vi "Main.vi"() -> ()   [LabVIEW 2024]
uses:
  Controls/Mode Enums/Bipolar Enum.ctl
  Controls/Activate Bools/Bipolar Activate Bool.ctl
  Controls/Plus-Minus Bools/Bipolar plus Bool.ctl
  Controls/Plus-Minus Bools/Bipolar minus Bool.ctl
  Controls/Activate Bools/Ligasure Activate Bool.ctl
  Controls/Mode Enums/Mono2 Coag Enum.ctl
  Controls/Activate Bools/Mono2 Coag Activate Bool.ctl
  Controls/Plus-Minus Bools/Mono2 Coag plus Bool.ctl
  Controls/Plus-Minus Bools/Mono2 Coag minus Bool.ctl
  Controls/Mode Enums/Mono2 Cut Enum.ctl
  Controls/Activate Bools/Mono2 Cut Activate Bool.ctl
  Controls/Plus-Minus Bools/Mono2 Cut plus Bool.ctl
  Controls/Plus-Minus Bools/Mono2 Cut minus Bool.ctl
  Controls/Mode Enums/Mono1 Coag Enum.ctl
  Controls/Activate Bools/Mono1 Coag Activate Bool.ctl
  Controls/Plus-Minus Bools/Mono1 Coag minus Bool.ctl
  Controls/Plus-Minus Bools/Mono1 Coag plus Bool.ctl
  Controls/Activate Bools/Mono1 Cut Activate Bool.ctl
  Controls/Mode Enums/Mono1 Cut Enum.ctl
  Controls/Plus-Minus Bools/Mono1 Cut plus Bool.ctl
  Controls/Plus-Minus Bools/Mono1 Cut minus Bool.ctl
  Controls/Tab Enums/Mono1 - Tab.ctl
  Controls/Tab Enums/Mono2 - Tab.ctl
  Controls/Activate Bools/Mono2 Triverse Activate Bool.ctl
  Controls/Tab Enums/Ligasure - Tab.ctl
  Controls/Tab Enums/Bipolar - Tab.ctl
  Controls/Cntrl - Power Bool.ctl
  Controls/QMH Fundamentals - Message Cluster.ctl
  Controls/Clusters/Message Handling Cluster.ctl
  Controls/Clusters/Control Handling Cluster.ctl
  Controls/Tab Enums/Activation Type Enum.ctl
  Controls/Clusters/Change Power Level Cluster.ctl
  Controls/Clusters/Activate Port Cluster.ctl
  Controls/Clusters/Change Mode Cluster.ctl
panel:
  in  "Show Graph":bool
  out "Display Message":string
  in  "Logging":bool
  in  "Power":T1
  in  "Main Tab":T2(tab)
  in  "CSV Test Path":path
  in  "Test Tab":enum32{"Run Test", "Edit Test"}(tab)
  in  "Abort Test":bool
  in  "Run Test":bool
  in  "Save CSV":bool
  in  "BldScript":i32[](listbox)
  in  "Load CSV":bool
  in  "Bipolar Enum":T3
  in  "Bipolar Activate":T4
  in  "Bipolar plus":T5
  in  "Bipolar minus":T6
  out "Bipolar Power":string
  in  "Ligasure Activate":T7
  in  "Mono2 Coag Enum":T8
  in  "Mono2 Coag Activate":T9
  in  "Mono2 Coag minus":T10
  in  "Mono2 Cut Enum":T11
  in  "Mono2 Cut Activate":T12
  in  "Mono2 Cut plus":T13
  in  "Mono2 Cut minus":T14
  out "Mono2 - Coag Power":string
  out "Mono2 - Cut Power":string
  in  "Mono2 Coag plus":T15
  in  "Mono1 Coag Enum":T16
  in  "Mono1 Coag Activate":T17
  in  "Mono1 Coag minus":T18
  in  "Mono1 Coag plus":T19
  out "Mono1 - Coag Power":string
  in  "Mono1 Cut Activate":T20
  out "Mono1 - Cut Power":string
  in  "Mono1 Cut Enum":T21
  in  "Mono1 Cut plus":T22
  in  "Mono1 Cut minus":T23
  in  "Mono1 - Tab":T24
  in  "Mono2 - Tab":T25
  in  "Mono2 Triverse Slide":i8(slide)=1 scale=1.0..5.0
  in  "Mono2 Triverse Activate":T26
  in  "Ligasure - Tab":T27
  in  "Bipolar - Tab":T28=enum."Auto Bipolar"
  in  "Connections Tab":T29(tab)
  in  "S2C Tab":enum32{"Build Script", "Execute Script"}(tab)
  in  "BldScript 2":i32[](listbox)
  in  "SubScript":string caption="SubScript Filename"
  in  "BldScriptFile":path caption="Test Script File"
  in  "BldBack":bool
  in  "BldLoadScript":bool
  in  "BldSaveScript":bool
  in  "BldSaveScriptAs":bool
  in  "BldClear":bool
  in  "ExeLoadScript":bool
  in  "ExeScriptFile":path caption="Script File"
  in  "ExeScript":i32[](listbox)
  in  "ExeExecute":bool
  in  "ExePause":bool
  in  "ExeNext":bool
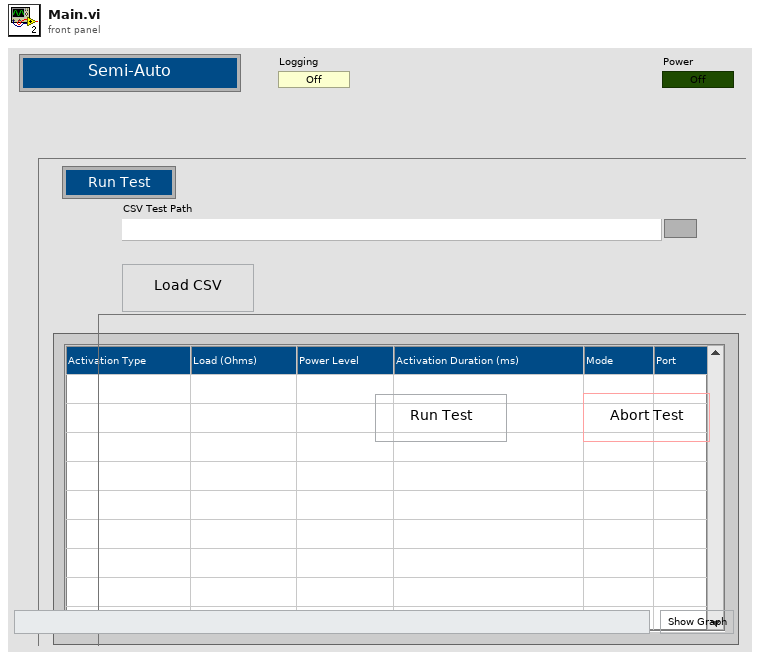
[diagram p1: front panel]
types:
  T1 = typedef "Cntrl - Power Bool.ctl" = bool
  T2 = enum32{"Semi-Auto", "Manual", "Connections", "Script 2 Code"}
  T3 = typedef "Bipolar Enum.ctl" = enum16{"Standard", "Macro", "Precision"}
  T4 = typedef "Bipolar Activate Bool.ctl" = bool
  T5 = typedef "Bipolar plus Bool.ctl" = bool
  T6 = typedef "Bipolar minus Bool.ctl" = bool
  T7 = typedef "Ligasure Activate Bool.ctl" = bool
  T8 = typedef "Mono2 Coag Enum.ctl" = enum16{"Spray", "Fulgerate"}
  T9 = typedef "Mono2 Coag Activate Bool.ctl" = bool
  T10 = typedef "Mono2 Coag minus Bool.ctl" = bool
  T11 = typedef "Mono2 Cut Enum.ctl" = enum16{"Pure", "Blend"}
  T12 = typedef "Mono2 Cut Activate Bool.ctl" = bool
  T13 = typedef "Mono2 Cut plus Bool.ctl" = bool
  T14 = typedef "Mono2 Cut minus Bool.ctl" = bool
  T15 = typedef "Mono2 Coag plus Bool.ctl" = bool
  T16 = typedef "Mono1 Coag Enum.ctl" = enum16{"Spray", "Fulgerate"}
  T17 = typedef "Mono1 Coag Activate Bool.ctl" = bool
  T18 = typedef "Mono1 Coag minus Bool.ctl" = bool
  T19 = typedef "Mono1 Coag plus Bool.ctl" = bool
  T20 = typedef "Mono1 Cut Activate Bool.ctl" = bool
  T21 = typedef "Mono1 Cut Enum.ctl" = enum16{"Pure", "Blend"}
  T22 = typedef "Mono1 Cut plus Bool.ctl" = bool
  T23 = typedef "Mono1 Cut minus Bool.ctl" = bool
  T24 = typedef "Mono1 - Tab.ctl" = enum32{"Mono1 - Fornax", "Mono1 - Handswitch", "Mono1 - Footswitch"}
  T25 = typedef "Mono2 - Tab.ctl" = enum32{"Mono2 - Fornax", "Mono2 - Handswitch", "Mono2 - Footswitch", "Mono2 - Triverse"}
  T26 = typedef "Mono2 Triverse Activate Bool.ctl" = bool
  T27 = typedef "Ligasure - Tab.ctl" = enum32{"Ligasure - Fornax", "Ligasure - Handswitch", "Ligasure - Footswitch"}
  T28 = typedef "Bipolar - Tab.ctl" = enum32{"Bipolar - Fornax", "Bipolar - Handswitch", "Bipolar - Footswitch", "Auto Bipolar"}
  T29 = enum32{"Digitizer Tab", "Fornax Tab", "FPGA Tab", "Nike Tab", "Relay Tab", "Rigel Tab"}
  T30 = typedef "Control Handling Cluster.ctl" = cluster{"Mono1 - Tab Enum":T31, "Mono2 - Tab Enum":T31, "Bipolar - Tab Enum":T31, "Ligasure - Tab Enum":T31}
  T31 = typedef "Activation Type Enum.ctl" = enum16{"Fornax", "Handswitch", "Footswitch", "Triverse", "Auto Bipolar"}
  T32 = typedef "Message Handling Cluster.ctl" = cluster{"Boolean":bool}
  T33 = typedef "QMH Fundamentals - Message Cluster.ctl" = cluster{"Message":string, "Message Data":variant}
  T34 = enum16{"Mono1 Cut", "Mono1 Coag", "Mono2 Cut", "Mono2 Coag", "Bipolar"}
  T35 = typedef "Change Power Level Cluster.ctl" = cluster{"Activation Type":enum16{"Mono1 Cut", "Mono1 Coag", "Mono2 Cut", "Mono2 Coag", "Bipolar"}, "Plus-Minus":enum16{"Plus", "Minus"}, "Plus-Minus":bool}
  T36 = enum16{"Mono1 Cut", "Mono1 Coag", "Mono2 Cut", "Mono2 Coag", "Mono2 Triverse", "Bipolar", "Ligasure"}
  T37 = typedef "Activate Port Cluster.ctl" = cluster{"Port":enum16{"Mono1 Cut", "Mono1 Coag", "Mono2 Cut", "Mono2 Coag", "Mono2 Triverse", "Bipolar", "Ligasure"}, "Activation Type Enum":T31, "Activate/Deactivate":bool}
  T38 = enum16{"Mono1 - Tab", "Mono2 - Tab", "Bipolar - Tab", "Ligasure - Tab"}
  T39 = enum32{"Invalid", "Standard", "Closed", "Hidden", "Minimized", "Maximized"}
  T40 = typedef "Change Mode Cluster.ctl" = cluster{"Port":enum16{"Mono1", "Mono2", "Bipolar", "Ligasure"}, "Mode":enum16{"Mono Pure", "Mono Blend", "Mono Fulgerate", "Mono Spray", "Bi Precision", "Bi Macro", "Bi Standard"}}
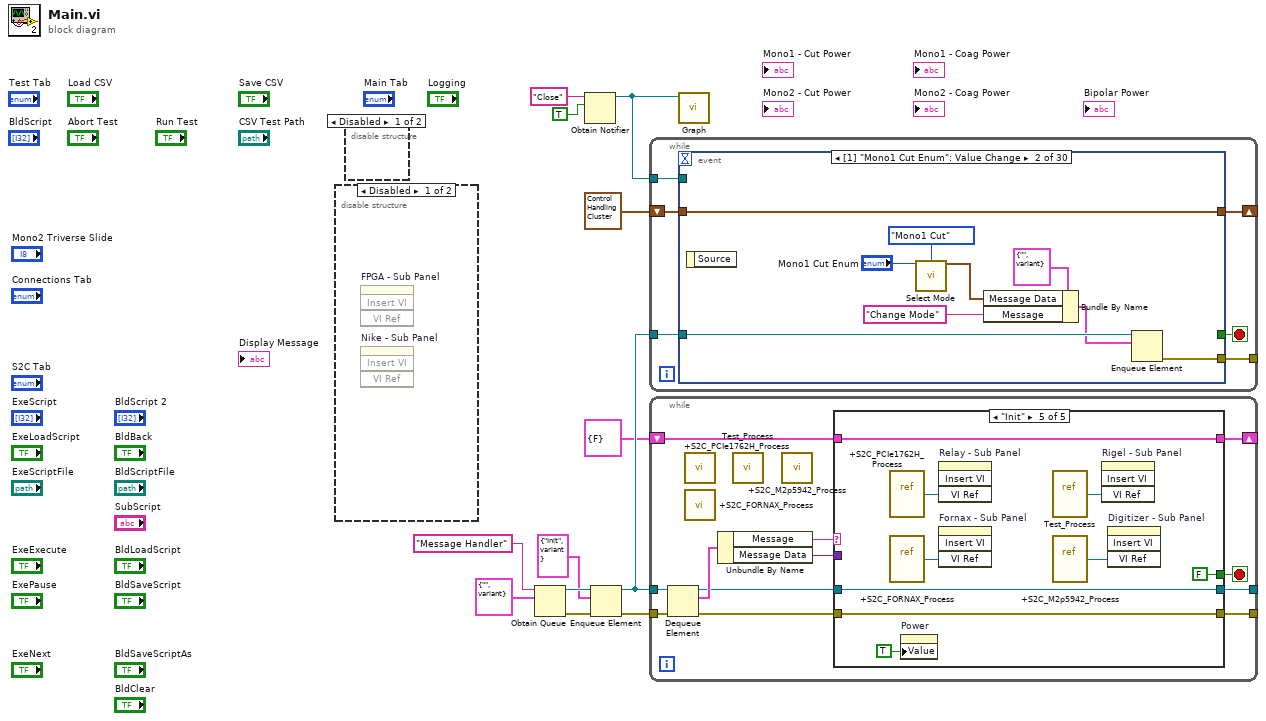
[diagram p0: block diagram]
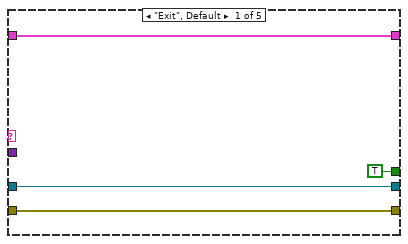
[diagram p4: hidden frame]
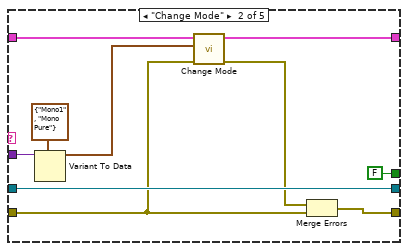
[diagram p5: hidden frame]
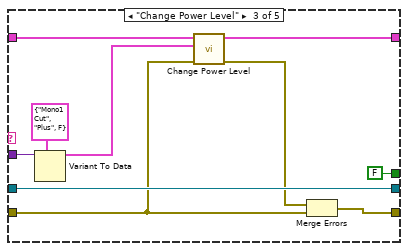
[diagram p6: hidden frame]
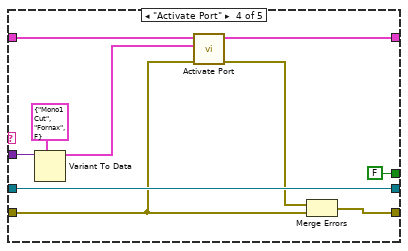
[diagram p7: hidden frame]
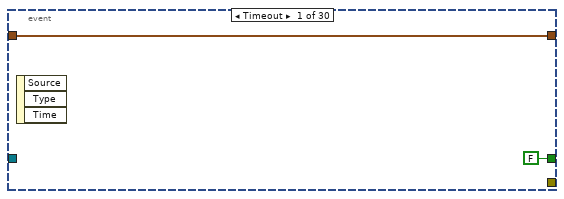
[diagram p8: hidden frame]
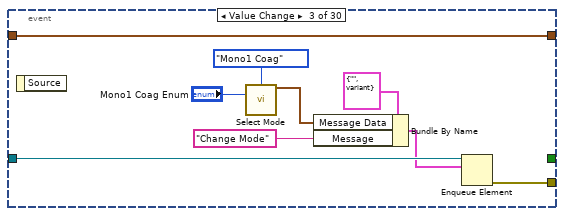
[diagram p9: hidden frame]
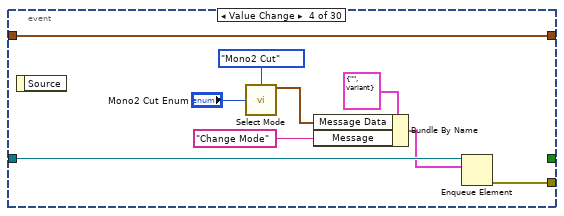
[diagram p10: hidden frame]
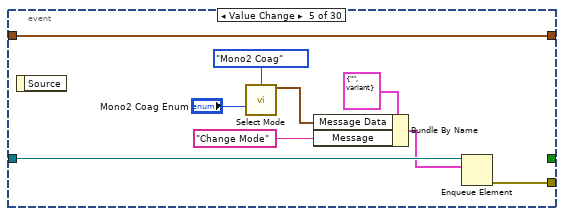
[diagram p11: hidden frame]
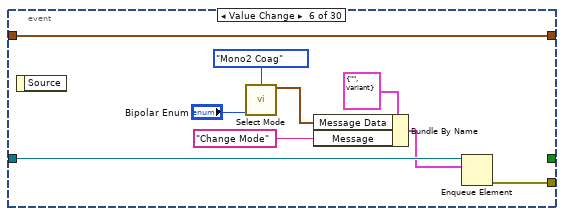
[diagram p12: hidden frame]
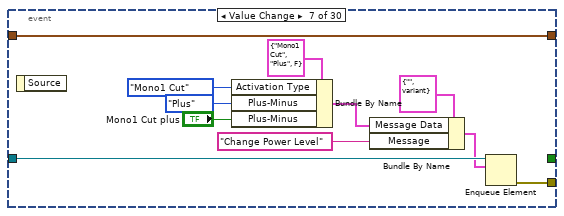
[diagram p13: hidden frame]
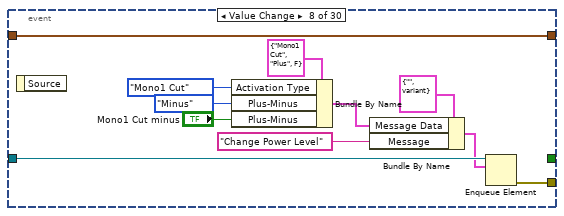
[diagram p14: hidden frame]
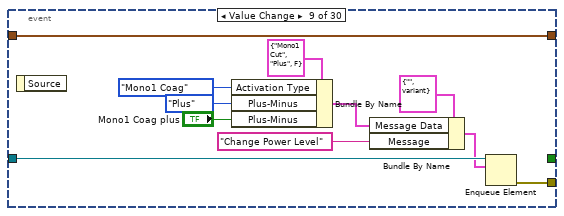
[diagram p15: hidden frame]
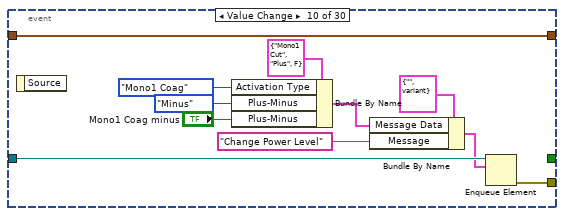
[diagram p16: hidden frame]
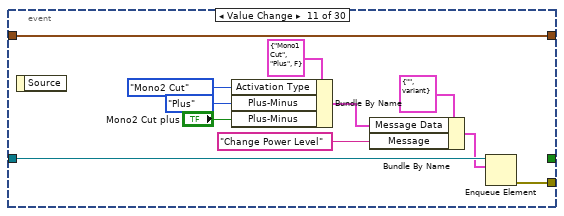
[diagram p17: hidden frame]
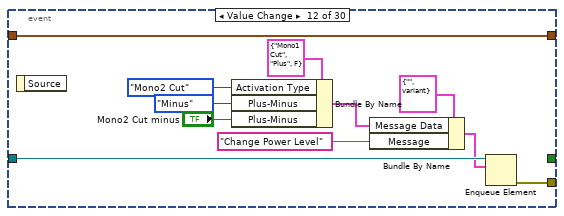
[diagram p18: hidden frame]
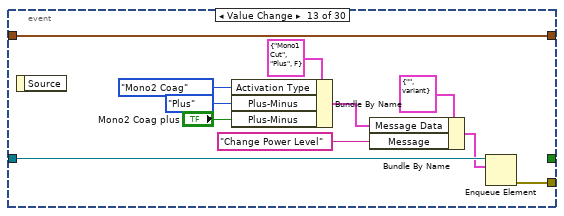
[diagram p19: hidden frame]
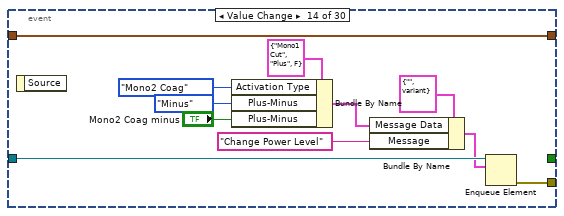
[diagram p20: hidden frame]
diagram:
  n1 = disable-structure shown="Disabled" {
    frame Disabled {
      n2 = invoke on="FPGA - Sub Panel" class="SubPnl" method="Insert VI"() -> ()  [unwired: 4 in, 4 out]
      n3 = invoke on="Nike - Sub Panel" class="SubPnl" method="Insert VI"() -> ()  [unwired: 4 in, 4 out]
    }
    frame Enabled {
    }
  }
  n4 = disable-structure shown="Disabled" {
    frame Disabled {
    }
    frame Enabled {
    }
  }
  n5 = Obtain Queue(name (unnamed)="Message Handler", element data type=T33 {"Message"="", "Message Data"=variant} ("Message Cluster")) -> (queue out=w11:refnum<queue>, error out=w12:errorcluster)  [unwired: 3 in, 1 out]
  n6 = Obtain Notifier(name (unnamed)="Close", notification data type=TRUE) -> (notifier out=w1:refnum<notifier>)  [unwired: 2 in, 2 out]
  n7 = Enqueue Element(queue=w11, element=T33 {"Message"="Init", "Message Data"=variant} ("Message Cluster"), error in (no error)=w12) -> (queue out=w6:refnum<queue>, error out=w9:errorcluster)  [unwired: 1 in, 1 out]
  n8 = while {
    tunnel: w6 -> [w17]
    tunnel: [w16] -> _
    shift-right: [w15] -> _
    shift-left: T30 {"Mono1 - Tab Enum"=enum."Fornax", "Mono2 - Tab Enum"=enum."Fornax", "Bipolar - Tab Enum"=enum."Fornax", "Ligasure - Tab Enum"=enum."Fornax"} ("Control Handling Cluster") -> [w14]
    tunnel: w1 -> [w13]
    stop <- w18 stop-if-true
    n9 = event shown="[1] \"Mono1 Cut Enum\": Value Change" {
      selector: _ -> [_ _ _ _ _ _ _ _ _ _ _ _ _ _ _ _ _ _ _ _ _ _ _ _ _ _ _ _ _ _]
      dyn-events: _ -> [_ _ _ _ _ _ _ _ _ _ _ _ _ _ _ _ _ _ _ _ _ _ _ _ _ _ _ _ _ _]
      timeout: _ -> [_ _ _ _ _ _ _ _ _ _ _ _ _ _ _ _ _ _ _ _ _ _ _ _ _ _ _ _ _ _]
      tunnel: [FALSE _ _ _ _ _ _ _ _ _ _ _ _ _ _ _ _ _ _ _ _ _ _ _ _ _ _ _ TRUE w286] -> w18
      tunnel: w17 -> [_ w29 w38 w47 w56 w65 w76 w87 w98 w109 w120 w131 w142 w153 w164 w175 w178 w190 w201 w212 w223 w234 w245 _ _ _ _ _ w285 w292]
      tunnel: [_ w26 w35 w44 w53 w62 w73 w84 w95 w106 w117 w128 w139 w150 w161 w172 w176 w188 w199 w210 w221 w232 w243 _ _ _ _ _ w283 w290] -> w16
      tunnel: [w19 w21 w30 w39 w48 w57 w71 w82 w93 w104 w115 w126 w137 w148 w159 w170 w185 w196 w207 w218 w229 w240 w251 w254 w260 w265 w270 w273 w281 w289] -> w15
      tunnel: w14 -> [w19 w21 w30 w39 w48 w57 w71 w82 w93 w104 w115 w126 w137 w148 w159 w170 w185 w196 w207 w218 w229 w240 w251 w257 w262 w267 w272 w273 w281 w289]
      tunnel: w13 -> [_ _ _ _ _ _ _ _ _ _ _ _ _ _ _ _ _ _ _ _ _ _ _ _ _ _ _ _ w279 w287]
      event Timeout {
        n10 = event-data() -> ()  [unwired: 1 in, 3 out]
      }
      event Value Change {
        n11 = event-data() -> ()  [unwired: 1 in, 1 out]
        n12 = call "Select Mode.vi"("Mono1 Cut Enum"="Mono1 Cut Enum", "Activation Type"=T34."Mono1 Cut") -> ("Change Mode Cluster"=w24:T40)  [unwired: 13 in]
        n13 = Bundle By Name(cluster=T33 {"Message"="", "Message Data"=variant} ("Message Cluster"), "Message Data"=w24, "Message"="Change Mode") -> (w27:T33)
        n14 = Enqueue Element(queue=w29, element=w27) -> (error out=w26:errorcluster)  [unwired: 2 in, 2 out]
      }
      event Value Change {
        n15 = event-data() -> ()  [unwired: 1 in, 1 out]
        n16 = call "Select Mode.vi"("Activation Type"=T34."Mono1 Coag", "Mono1 Coag Enum"="Mono1 Coag Enum") -> ("Change Mode Cluster"=w33:T40)  [unwired: 13 in]
        n17 = Bundle By Name(cluster=T33 {"Message"="", "Message Data"=variant} ("Message Cluster"), "Message Data"=w33, "Message"="Change Mode") -> (w36:T33)
        n18 = Enqueue Element(queue=w38, element=w36) -> (error out=w35:errorcluster)  [unwired: 2 in, 2 out]
      }
      event Value Change {
        n19 = event-data() -> ()  [unwired: 1 in, 1 out]
        n20 = call "Select Mode.vi"("Activation Type"=T34."Mono2 Cut", "Mono2 Cut Enum"="Mono2 Cut Enum") -> ("Change Mode Cluster"=w42:T40)  [unwired: 13 in]
        n21 = Bundle By Name(cluster=T33 {"Message"="", "Message Data"=variant} ("Message Cluster"), "Message Data"=w42, "Message"="Change Mode") -> (w45:T33)
        n22 = Enqueue Element(queue=w47, element=w45) -> (error out=w44:errorcluster)  [unwired: 2 in, 2 out]
      }
      event Value Change {
        n23 = event-data() -> ()  [unwired: 1 in, 1 out]
        n24 = call "Select Mode.vi"("Activation Type"=T34."Mono2 Coag", "Mono2 Coag Enum"="Mono2 Coag Enum") -> ("Change Mode Cluster"=w51:T40)  [unwired: 13 in]
        n25 = Bundle By Name(cluster=T33 {"Message"="", "Message Data"=variant} ("Message Cluster"), "Message Data"=w51, "Message"="Change Mode") -> (w54:T33)
        n26 = Enqueue Element(queue=w56, element=w54) -> (error out=w53:errorcluster)  [unwired: 2 in, 2 out]
      }
      event Value Change {
        n27 = event-data() -> ()  [unwired: 1 in, 1 out]
        n28 = call "Select Mode.vi"("Activation Type"=T34."Mono2 Coag", "Bipolar Enum"="Bipolar Enum") -> ("Change Mode Cluster"=w60:T40)  [unwired: 13 in]
        n29 = Bundle By Name(cluster=T33 {"Message"="", "Message Data"=variant} ("Message Cluster"), "Message Data"=w60, "Message"="Change Mode") -> (w63:T33)
        n30 = Enqueue Element(queue=w65, element=w63) -> (error out=w62:errorcluster)  [unwired: 2 in, 2 out]
      }
      event Value Change {
        n31 = event-data() -> ()  [unwired: 1 in, 1 out]
        n32 = Bundle By Name(cluster=T35 {"Activation Type"=enum."Mono1 Cut", "Plus-Minus"=enum."Plus", "Plus-Minus"=FALSE}, "Activation Type"=T34."Mono1 Cut", "Plus-Minus"=enum16{"Plus", "Minus"}."Plus", "Plus-Minus"="Mono1 Cut plus") -> (w67:T35)
        n33 = Bundle By Name(cluster=T33 {"Message"="", "Message Data"=variant} ("Message Cluster"), "Message Data"=w67, "Message"="Change Power Level") -> (w74:T33)
        n34 = Enqueue Element(queue=w76, element=w74) -> (error out=w73:errorcluster)  [unwired: 2 in, 2 out]
      }
      event Value Change {
        n35 = event-data() -> ()  [unwired: 1 in, 1 out]
        n36 = Bundle By Name(cluster=T35 {"Activation Type"=enum."Mono1 Cut", "Plus-Minus"=enum."Plus", "Plus-Minus"=FALSE}, "Activation Type"=T34."Mono1 Cut", "Plus-Minus"=enum16{"Plus", "Minus"}."Minus", "Plus-Minus"="Mono1 Cut minus") -> (w78:T35)
        n37 = Bundle By Name(cluster=T33 {"Message"="", "Message Data"=variant} ("Message Cluster"), "Message Data"=w78, "Message"="Change Power Level") -> (w85:T33)
        n38 = Enqueue Element(queue=w87, element=w85) -> (error out=w84:errorcluster)  [unwired: 2 in, 2 out]
      }
      event Value Change {
        n39 = event-data() -> ()  [unwired: 1 in, 1 out]
        n40 = Bundle By Name(cluster=T35 {"Activation Type"=enum."Mono1 Cut", "Plus-Minus"=enum."Plus", "Plus-Minus"=FALSE}, "Activation Type"=T34."Mono1 Coag", "Plus-Minus"=enum16{"Plus", "Minus"}."Plus", "Plus-Minus"="Mono1 Coag plus") -> (w89:T35)
        n41 = Bundle By Name(cluster=T33 {"Message"="", "Message Data"=variant} ("Message Cluster"), "Message Data"=w89, "Message"="Change Power Level") -> (w96:T33)
        n42 = Enqueue Element(queue=w98, element=w96) -> (error out=w95:errorcluster)  [unwired: 2 in, 2 out]
      }
      event Value Change {
        n43 = event-data() -> ()  [unwired: 1 in, 1 out]
        n44 = Bundle By Name(cluster=T35 {"Activation Type"=enum."Mono1 Cut", "Plus-Minus"=enum."Plus", "Plus-Minus"=FALSE}, "Activation Type"=T34."Mono1 Coag", "Plus-Minus"=enum16{"Plus", "Minus"}."Minus", "Plus-Minus"="Mono1 Coag minus") -> (w100:T35)
        n45 = Bundle By Name(cluster=T33 {"Message"="", "Message Data"=variant} ("Message Cluster"), "Message Data"=w100, "Message"="Change Power Level") -> (w107:T33)
        n46 = Enqueue Element(queue=w109, element=w107) -> (error out=w106:errorcluster)  [unwired: 2 in, 2 out]
      }
      event Value Change {
        n47 = event-data() -> ()  [unwired: 1 in, 1 out]
        n48 = Bundle By Name(cluster=T35 {"Activation Type"=enum."Mono1 Cut", "Plus-Minus"=enum."Plus", "Plus-Minus"=FALSE}, "Activation Type"=T34."Mono2 Cut", "Plus-Minus"=enum16{"Plus", "Minus"}."Plus", "Plus-Minus"="Mono2 Cut plus") -> (w111:T35)
        n49 = Bundle By Name(cluster=T33 {"Message"="", "Message Data"=variant} ("Message Cluster"), "Message Data"=w111, "Message"="Change Power Level") -> (w118:T33)
        n50 = Enqueue Element(queue=w120, element=w118) -> (error out=w117:errorcluster)  [unwired: 2 in, 2 out]
      }
      event Value Change {
        n51 = event-data() -> ()  [unwired: 1 in, 1 out]
        n52 = Bundle By Name(cluster=T35 {"Activation Type"=enum."Mono1 Cut", "Plus-Minus"=enum."Plus", "Plus-Minus"=FALSE}, "Activation Type"=T34."Mono2 Cut", "Plus-Minus"=enum16{"Plus", "Minus"}."Minus", "Plus-Minus"="Mono2 Cut minus") -> (w122:T35)
        n53 = Bundle By Name(cluster=T33 {"Message"="", "Message Data"=variant} ("Message Cluster"), "Message Data"=w122, "Message"="Change Power Level") -> (w129:T33)
        n54 = Enqueue Element(queue=w131, element=w129) -> (error out=w128:errorcluster)  [unwired: 2 in, 2 out]
      }
      event Value Change {
        n55 = event-data() -> ()  [unwired: 1 in, 1 out]
        n56 = Bundle By Name(cluster=T35 {"Activation Type"=enum."Mono1 Cut", "Plus-Minus"=enum."Plus", "Plus-Minus"=FALSE}, "Activation Type"=T34."Mono2 Coag", "Plus-Minus"=enum16{"Plus", "Minus"}."Plus", "Plus-Minus"="Mono2 Coag plus") -> (w133:T35)
        n57 = Bundle By Name(cluster=T33 {"Message"="", "Message Data"=variant} ("Message Cluster"), "Message Data"=w133, "Message"="Change Power Level") -> (w140:T33)
        n58 = Enqueue Element(queue=w142, element=w140) -> (error out=w139:errorcluster)  [unwired: 2 in, 2 out]
      }
      event Value Change {
        n59 = event-data() -> ()  [unwired: 1 in, 1 out]
        n60 = Bundle By Name(cluster=T35 {"Activation Type"=enum."Mono1 Cut", "Plus-Minus"=enum."Plus", "Plus-Minus"=FALSE}, "Activation Type"=T34."Mono2 Coag", "Plus-Minus"=enum16{"Plus", "Minus"}."Minus", "Plus-Minus"="Mono2 Coag minus") -> (w144:T35)
        n61 = Bundle By Name(cluster=T33 {"Message"="", "Message Data"=variant} ("Message Cluster"), "Message Data"=w144, "Message"="Change Power Level") -> (w151:T33)
        n62 = Enqueue Element(queue=w153, element=w151) -> (error out=w150:errorcluster)  [unwired: 2 in, 2 out]
      }
      event Value Change {
        n63 = event-data() -> ()  [unwired: 1 in, 1 out]
        n64 = Bundle By Name(cluster=T35 {"Activation Type"=enum."Mono1 Cut", "Plus-Minus"=enum."Plus", "Plus-Minus"=FALSE}, "Activation Type"=T34."Bipolar", "Plus-Minus"=enum16{"Plus", "Minus"}."Plus", "Plus-Minus"="Bipolar plus") -> (w155:T35)
        n65 = Bundle By Name(cluster=T33 {"Message"="", "Message Data"=variant} ("Message Cluster"), "Message Data"=w155, "Message"="Change Power Level") -> (w162:T33)
        n66 = Enqueue Element(queue=w164, element=w162) -> (error out=w161:errorcluster)  [unwired: 2 in, 2 out]
      }
      event Value Change {
        n67 = event-data() -> ()  [unwired: 1 in, 1 out]
        n68 = Bundle By Name(cluster=T35 {"Activation Type"=enum."Mono1 Cut", "Plus-Minus"=enum."Plus", "Plus-Minus"=FALSE}, "Activation Type"=T34."Bipolar", "Plus-Minus"=enum16{"Plus", "Minus"}."Minus", "Plus-Minus"="Bipolar minus") -> (w166:T35)
        n69 = Bundle By Name(cluster=T33 {"Message"="", "Message Data"=variant} ("Message Cluster"), "Message Data"=w166, "Message"="Change Power Level") -> (w173:T33)
        n70 = Enqueue Element(queue=w175, element=w173) -> (error out=w172:errorcluster)  [unwired: 2 in, 2 out]
      }
      event Value Change {
        n71 = event-data() -> ()  [unwired: 1 in, 1 out]
        n72 = Unbundle By Name(w185) -> ("Mono1 - Tab Enum"=w184:T31)
        n73 = Bundle By Name(cluster=T37 {"Port"=enum."Mono1 Cut", "Activation Type Enum"=enum."Fornax", "Activate/Deactivate"=FALSE}, "Activation Type Enum"=w184, "Port"=T36."Mono1 Cut", "Activate/Deactivate"="Mono1 Cut Activate") -> (w177:T37)
        n74 = Bundle By Name(cluster=T33 {"Message"="", "Message Data"=variant} ("Message Cluster"), "Message Data"=w177, "Message"="Activate Port") -> (w180:T33)
        n75 = Enqueue Element(queue=w178, element=w180) -> (error out=w176:errorcluster)  [unwired: 2 in, 2 out]
      }
      event Value Change {
        n76 = event-data() -> ()  [unwired: 1 in, 1 out]
        n77 = Unbundle By Name(w196) -> ("Mono1 - Tab Enum"=w195:T31)
        n78 = Bundle By Name(cluster=T37 {"Port"=enum."Mono1 Cut", "Activation Type Enum"=enum."Fornax", "Activate/Deactivate"=FALSE}, "Activation Type Enum"=w195, "Port"=T36."Mono1 Coag", "Activate/Deactivate"="Mono1 Coag Activate") -> (w189:T37)
        n79 = Bundle By Name(cluster=T33 {"Message"="", "Message Data"=variant} ("Message Cluster"), "Message Data"=w189, "Message"="Activate Port") -> (w192:T33)
        n80 = Enqueue Element(queue=w190, element=w192) -> (error out=w188:errorcluster)  [unwired: 2 in, 2 out]
      }
      event Value Change {
        n81 = event-data() -> ()  [unwired: 1 in, 1 out]
        n82 = Unbundle By Name(w207) -> ("Mono2 - Tab Enum"=w206:T31)
        n83 = Bundle By Name(cluster=T37 {"Port"=enum."Mono1 Cut", "Activation Type Enum"=enum."Fornax", "Activate/Deactivate"=FALSE}, "Activation Type Enum"=w206, "Port"=T36."Mono2 Cut", "Activate/Deactivate"="Mono2 Cut Activate") -> (w200:T37)
        n84 = Bundle By Name(cluster=T33 {"Message"="", "Message Data"=variant} ("Message Cluster"), "Message Data"=w200, "Message"="Activate Port") -> (w203:T33)
        n85 = Enqueue Element(queue=w201, element=w203) -> (error out=w199:errorcluster)  [unwired: 2 in, 2 out]
      }
      event Value Change {
        n86 = event-data() -> ()  [unwired: 1 in, 1 out]
        n87 = Unbundle By Name(w218) -> ("Mono2 - Tab Enum"=w217:T31)
        n88 = Bundle By Name(cluster=T37 {"Port"=enum."Mono1 Cut", "Activation Type Enum"=enum."Fornax", "Activate/Deactivate"=FALSE}, "Activation Type Enum"=w217, "Port"=T36."Mono2 Coag", "Activate/Deactivate"="Mono2 Coag Activate") -> (w211:T37)
        n89 = Bundle By Name(cluster=T33 {"Message"="", "Message Data"=variant} ("Message Cluster"), "Message Data"=w211, "Message"="Activate Port") -> (w214:T33)
        n90 = Enqueue Element(queue=w212, element=w214) -> (error out=w210:errorcluster)  [unwired: 2 in, 2 out]
      }
      event Value Change {
        n91 = event-data() -> ()  [unwired: 1 in, 1 out]
        n92 = Unbundle By Name(w229) -> ("Mono2 - Tab Enum"=w228:T31)
        n93 = Bundle By Name(cluster=T37 {"Port"=enum."Mono1 Cut", "Activation Type Enum"=enum."Fornax", "Activate/Deactivate"=FALSE}, "Activation Type Enum"=w228, "Port"=T36."Mono2 Triverse", "Activate/Deactivate"="Mono2 Triverse Activate") -> (w222:T37)
        n94 = Bundle By Name(cluster=T33 {"Message"="", "Message Data"=variant} ("Message Cluster"), "Message Data"=w222, "Message"="Activate Port") -> (w225:T33)
        n95 = Enqueue Element(queue=w223, element=w225) -> (error out=w221:errorcluster)  [unwired: 2 in, 2 out]
      }
      event Value Change {
        n96 = event-data() -> ()  [unwired: 1 in, 1 out]
        n97 = Unbundle By Name(w240) -> ("Bipolar - Tab Enum"=w239:T31)
        n98 = Bundle By Name(cluster=T37 {"Port"=enum."Mono1 Cut", "Activation Type Enum"=enum."Fornax", "Activate/Deactivate"=FALSE}, "Activation Type Enum"=w239, "Port"=T36."Bipolar", "Activate/Deactivate"="Bipolar Activate") -> (w233:T37)
        n99 = Bundle By Name(cluster=T33 {"Message"="", "Message Data"=variant} ("Message Cluster"), "Message Data"=w233, "Message"="Activate Port") -> (w236:T33)
        n100 = Enqueue Element(queue=w234, element=w236) -> (error out=w232:errorcluster)  [unwired: 2 in, 2 out]
      }
      event Value Change {
        n101 = event-data() -> ()  [unwired: 1 in, 1 out]
        n102 = Unbundle By Name(w251) -> ("Ligasure - Tab Enum"=w250:T31)
        n103 = Bundle By Name(cluster=T37 {"Port"=enum."Mono1 Cut", "Activation Type Enum"=enum."Fornax", "Activate/Deactivate"=FALSE}, "Activation Type Enum"=w250, "Port"=T36."Ligasure", "Activate/Deactivate"="Ligasure Activate") -> (w244:T37)
        n104 = Bundle By Name(cluster=T33 {"Message"="", "Message Data"=variant} ("Message Cluster"), "Message Data"=w244, "Message"="Activate Port") -> (w247:T33)
        n105 = Enqueue Element(queue=w245, element=w247) -> (error out=w243:errorcluster)  [unwired: 2 in, 2 out]
      }
      event Value Change {
        n106 = event-data() -> ()  [unwired: 1 in, 1 out]
        n107 = call "Change Activation Type.vi"("Tab Selector"=T38."Mono1 - Tab", "Mono1 - Tab"="Mono1 - Tab") -> ("Mono1 - Tab Enum"=w253:T31)  [unwired: 6 in, 3 out]
        n108 = Bundle By Name(cluster=w257, "Mono1 - Tab Enum"=w253) -> (w254:T30)
      }
      event Value Change {
        n109 = event-data() -> ()  [unwired: 1 in, 1 out]
        n110 = call "Change Activation Type.vi"("Tab Selector"=T38."Mono2 - Tab", "Mono2 - Tab"="Mono2 - Tab") -> ("Mono2 - Tab Enum"=w258:T31)  [unwired: 6 in, 3 out]
        n111 = Bundle By Name(cluster=w262, "Mono2 - Tab Enum"=w258) -> (w260:T30)
      }
      event Value Change {
        n112 = event-data() -> ()  [unwired: 1 in, 1 out]
        n113 = call "Change Activation Type.vi"("Tab Selector"=T38."Bipolar - Tab", "Bipolar - Tab"="Bipolar - Tab") -> ("Bipolar - Tab Enum"=w263:T31)  [unwired: 6 in, 3 out]
        n114 = Bundle By Name(cluster=w267, "Bipolar - Tab Enum"=w263) -> (w265:T30)
      }
      event Value Change {
        n115 = event-data() -> ()  [unwired: 1 in, 1 out]
        n116 = call "Change Activation Type.vi"("Tab Selector"=T38."Ligasure - Tab", "Ligasure - Tab"="Ligasure - Tab") -> ("Ligasure - Tab Enum"=w268:T31)  [unwired: 6 in, 3 out]
        n117 = Bundle By Name(cluster=w272, "Ligasure - Tab Enum"=w268) -> (w270:T30)
      }
      event "Show Graph": Value Change {
        n118 = event-data() -> ()  [unwired: 1 in, 1 out]
        n119 = Select(t=T39."Standard" ("State"), s="Show Graph", f=T39."Hidden" ("State")) -> (s? t:f=w274:T39)
        n120 = vi-ref "Graph.vi"() -> (w278:refnum<vi>)
        n121 = invoke class="VI" method="FP.Open"(reference=w278, "State"=w274) -> ()  [unwired: 3 in, 5 out]
      }
      event Value Change {
        n122 = event-data() -> ()  [unwired: 1 in, 1 out]
        n123 = Send Notification(notification=TRUE, notifier=w279) -> ()  [unwired: 1 in, 2 out]
        n124 = Enqueue Element At Opposite End(queue=w285, element=T33 {"Message"="Exit", "Message Data"=variant} ("Message Cluster")) -> (error out=w283:errorcluster)  [unwired: 2 in, 2 out]
      }
      event Panel Close? {
        w286 = TRUE
        n125 = event-data() -> ()  [unwired: 1 in, 1 out]
        n126 = Send Notification(notification=TRUE, notifier=w287) -> ()  [unwired: 1 in, 2 out]
        n127 = Enqueue Element At Opposite End(queue=w292, element=T33 {"Message"="Exit", "Message Data"=variant} ("Message Cluster")) -> (error out=w290:errorcluster)  [unwired: 2 in, 2 out]
        n128 = event-data("Discard?"=w286) -> ()  [unwired: 1 in, 1 out]
      }
    }
  }
  n129 = while {
    tunnel: w6 -> [w303]
    tunnel: w9 -> [w302]
    tunnel: [w297] -> _
    tunnel: [w296] -> _
    shift-right: [w294] -> _
    shift-left: T32 {"Boolean"=FALSE} -> [w293]
    stop <- w295 stop-if-true
    n130 = Dequeue Element(queue=w303, error in (no error)=w302) -> (queue out=w299:refnum<queue>, element=w304:T33, error out=w298:errorcluster)  [unwired: 1 in, 1 out]
    n131 = call "+S2C_PCIe1762H_Process.vi"() -> ()  [unwired: 11 in, 1 out]
    n132 = call "+S2C_FORNAX_Process.vi"() -> ()  [unwired: 11 in, 1 out]
    n133 = Unbundle By Name(w304) -> ("Message"=w301:string, "Message Data"=w300:variant)
    n134 = call "Test_Process.vi"() -> ()  [unwired: 11 in, 1 out]
    n135 = call "+S2C_M2p5942_Process.vi"() -> ()  [unwired: 11 in, 1 out]
    n136 = case shown="\"Init\"" w301 {
      tunnel: w300 -> [_ w316 w326 w336 _]
      tunnel: w299 -> [w308 w318 w328 w338 w347]
      tunnel: w298 -> [w307 w311 w321 w333 w346]
      tunnel: [w308 w318 w328 w338 w347] -> w297
      tunnel: [w307 w310 w325 w335 w346] -> w296
      tunnel: [TRUE FALSE FALSE FALSE FALSE] -> w295
      tunnel: [w305 w312 w319 w330 w343] -> w294
      tunnel: w293 -> [w305 w313 w323 w331 w343]
      frame "Exit", Default {
      }
      frame "Change Mode" {
        n137 = Variant To Data(type=T40 {"Port"=enum."Mono1", "Mode"=enum."Mono Pure"}, Variant=w316) -> (data=w314:T40)  [unwired: 1 in, 1 out]
        n138 = call "Change Mode.vi"("error in"=w311, "Change Mode Cluster"=w314, "Message Handling Cluster in"=w313) -> ("error out"=w309:errorcluster, "Message Handling Cluster out"=w312:T32)  [unwired: 7 in]
        n139 = Merge Errors(w309, w311) -> (w310:errorcluster)
      }
      frame "Change Power Level" {
        n140 = Variant To Data(type=T35 {"Activation Type"=enum."Mono1 Cut", "Plus-Minus"=enum."Plus", "Plus-Minus"=FALSE}, Variant=w326) -> (data=w322:T35)  [unwired: 1 in, 1 out]
        n141 = call "Change Power Level.vi"("error in (no error)"=w321, "Change Power Level Cluster"=w322, "Message Handling Cluster in"=w323) -> ("error out"=w320:errorcluster, "Message Handling Cluster out"=w319:T32)  [unwired: 7 in]
        n142 = Merge Errors(w320, w321) -> (w325:errorcluster)
      }
      frame "Activate Port" {
        n143 = Variant To Data(type=T37 {"Port"=enum."Mono1 Cut", "Activation Type Enum"=enum."Fornax", "Activate/Deactivate"=FALSE}, Variant=w336) -> (data=w329:T37)  [unwired: 1 in, 1 out]
        n144 = call "Activate Port.vi"("error in (no error)"=w333, "data"=w329, "Message Handling Cluster"=w331) -> ("error out"=w332:errorcluster, "Message Handling Cluster"=w330:T32)  [unwired: 7 in]
        n145 = Merge Errors(w332, w333) -> (w335:errorcluster)
      }
      frame "Init" {
        n146 = vi-ref "+S2C_PCIe1762H_Process.vi"() -> (w340:refnum<vi>)
        n147 = vi-ref "+S2C_FORNAX_Process.vi"() -> (w339:refnum<vi>)
        n148 = property on="Power" class="Bool (strict)"("Value"=T1 TRUE ("Power")) -> ()  [unwired: 2 in, 2 out]
        n149 = invoke on="Relay - Sub Panel" class="SubPnl" method="Insert VI"("VI Ref"=w340) -> ()  [unwired: 3 in, 4 out]
        n150 = invoke on="Fornax - Sub Panel" class="SubPnl" method="Insert VI"("VI Ref"=w339) -> ()  [unwired: 3 in, 4 out]
        n151 = vi-ref "Test_Process.vi"() -> (w342:refnum<vi>)
        n152 = vi-ref "+S2C_M2p5942_Process.vi"() -> (w341:refnum<vi>)
        n153 = invoke on="Rigel - Sub Panel" class="SubPnl" method="Insert VI"("VI Ref"=w342) -> ()  [unwired: 3 in, 4 out]
        n154 = invoke on="Digitizer - Sub Panel" class="SubPnl" method="Insert VI"("VI Ref"=w341) -> ()  [unwired: 3 in, 4 out]
      }
    }
  }
  n155 = call "Graph.vi"("Notifier in"=w1) -> ()  [unwired: 11 in]
